vi "G4SubTemplate_Singleton_4x4x4_GetProperty.vi"(8 "Error In":errorcluster) -> (0 "Error Out":errorcluster, 2 "Property":dbl)   [LabVIEW 2020]
uses:
  <resource>/Framework/Providers/Open_GDS/ClassProviders/Provider_EndevoGOOP400/Templates/G4SubTemplate_Singleton_4x4x4/G4SubTemplate_Singleton_4x4x4.lvclass
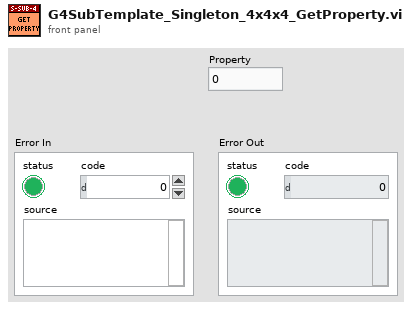
[diagram p1: front panel]
types:
  T1 = typedef "G4SubTemplate_Singleton_4x4x4.lvclass/ObjectAttributes.ctl" = cluster{"Attribute1":dbl}
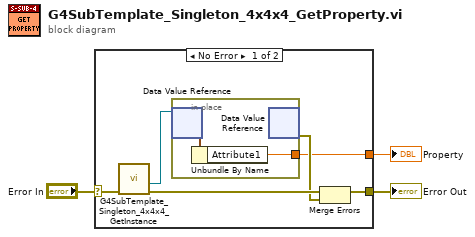
[diagram p0: block diagram]
diagram:
  n1 = case shown="No Error" "Error In" {
    selector: "Error In" -> [w9 w12]
    tunnel: [w7 w12] -> w2
    tunnel: [w5 _] -> w1
    frame No Error {
      n2 = call <resource>:"G4SubTemplate_Singleton_4x4x4_GetInstance.vi"("error in"=w9) -> ("error out"=w8:errorcluster, "DVRRefOut"=w4:refnum<data-value>)  [unwired: 6 in, 3 out]
      n3 = in-place {
        in-place-border: [w11] -> w5
        n4 = in-place-dvr #1(w4) -> (w10:T1)  [unwired: 1 out]
        n5 = Unbundle By Name(w10) -> ("Attribute1"=w11:dbl)
        n6 = in-place-dvr #1() -> (w6:errorcluster)  [unwired: 1 in, 1 out]
      }
      n7 = Merge Errors(w8, w6) -> (w7:errorcluster)
    }
    frame Error {
    }
  }
  "Error Out" <- w2
  "Property" <- w1
